vi "SIM Registry Register Node (vector).vi"(0 "Registry In":T1, 5 "Has ZC?":bool, 9 "Output Width":i32=-1, 11 "Input Width":i32=-1, 14 "Tag":string) -> (4 "Registry Out":T1, 6 "Block Idx":i32)   [LabVIEW 2020]
uses:
  <vilib>/Simulation/Implementation/Shared/SIM Registry.llb/SIM Simulation Registry.ctl
  <vilib>/Simulation/Implementation/Shared/SIM Registry.llb/SIM Registry Node Header.ctl
  <vilib>/Simulation/Implementation/Shared/SIM Registry.llb/SIM Registry Node Record.ctl
  <vilib>/Simulation/Implementation/Shared/SIM trigger type.ctl
  <vilib>/Simulation/Implementation/Shared/SIM solver state data.ctl
  <vilib>/Simulation/Implementation/Shared/SIM limit type.ctl
  <vilib>/Simulation/Implementation/Shared/SIM discrete data.ctl
  <vilib>/Simulation/Implementation/Shared/SIM Discrete state data.ctl
  <vilib>/Simulation/Implementation/Shared/SIM Registry.llb/SIM Simulation Registry Error.ctl
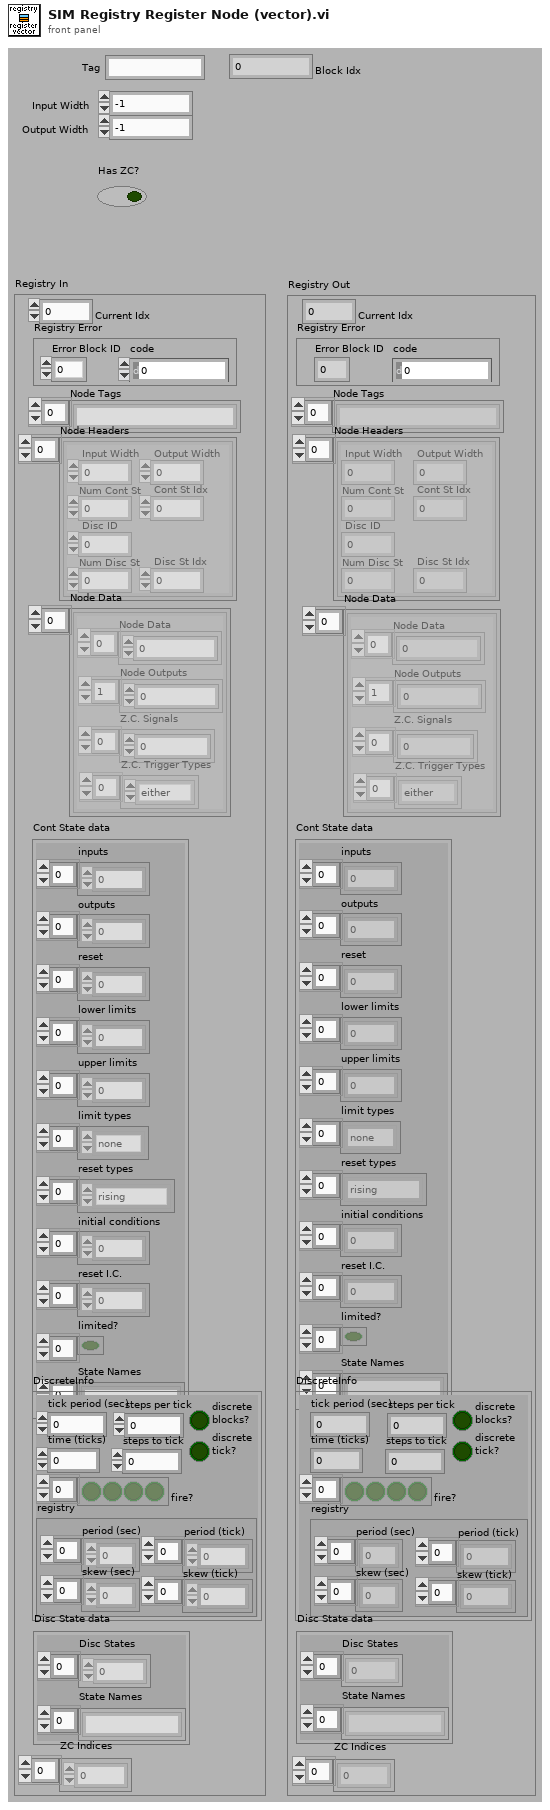
[diagram p1: front panel]
types:
  T1 = typedef "SIM Simulation Registry.ctl" = cluster{"Current Idx":i32, "Node Tags":string[], "Node Headers":T2[], "Node Data":T3[], "Cont State data":T5, "DiscreteInfo":T7, "Disc State data":T8, "Registry Error":T9, "ZC Indices":i32[]}
  T2 = typedef "SIM Registry Node Header.ctl" = cluster{"Input Width":i32, "Disc ID":i32, "Num Cont St":i32, "Cont St Idx":i32, "Num Disc St":i32, "Disc St Idx":i32, "Output Width":i32}
  T3 = typedef "SIM Registry Node Record.ctl" = cluster{"Node Data":dbl[], "Node Outputs":dbl[], "Z.C. Signals":dbl[], "Z.C. Trigger Types":T4[]}
  T4 = typedef "SIM trigger type.ctl" = enum16{"rising", "falling", "either", "none"}
  T5 = typedef "SIM solver state data.ctl" = cluster{"inputs":dbl[], "outputs":dbl[], "reset":dbl[], "lower limits":dbl[], "upper limits":dbl[], "limit types":T6[], "reset types":T4[], "initial conditions":dbl[], "reset I.C.":dbl[], "limited?":bool[], "State Names":string[]}
  T6 = typedef "SIM limit type.ctl" = enum16{"upper", "lower", "both", "none"}
  T7 = typedef "SIM discrete data.ctl" = cluster{"tick period (sec)":dbl, "time (ticks)":i32, "fire?":bool[], "registry":cluster{"period (sec)":dbl[], "skew (sec)":dbl[], "period (tick)":i32[], "skew (tick)":i32[]}, "discrete \nblocks?":bool, "steps per tick":dbl, "steps to tick":dbl, "discrete \ntick?":bool}
  T8 = typedef "SIM Discrete state data.ctl" = cluster{"Disc States":dbl[], "State Names":string[]}
  T9 = typedef "SIM Simulation Registry Error.ctl" = cluster{"Error Block ID":i32, "code":i32}
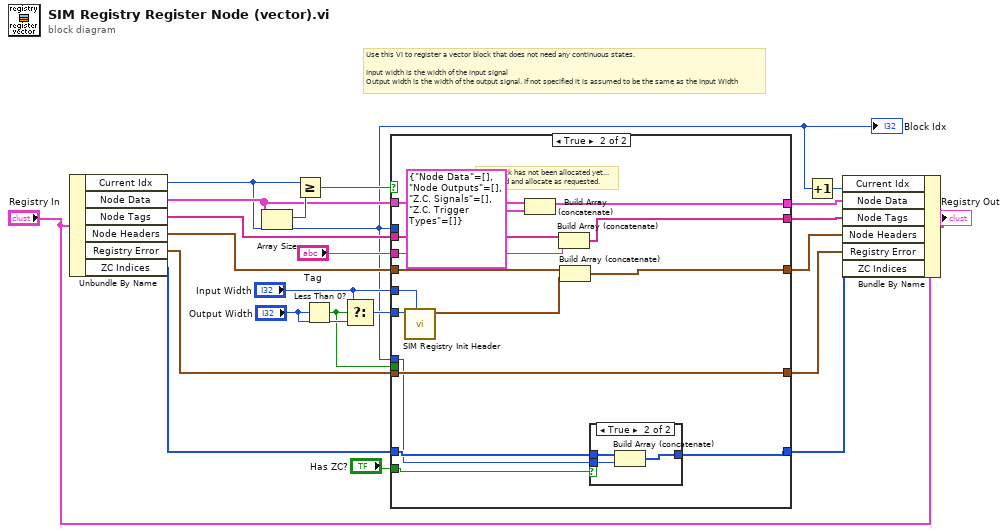
[diagram p0: block diagram]
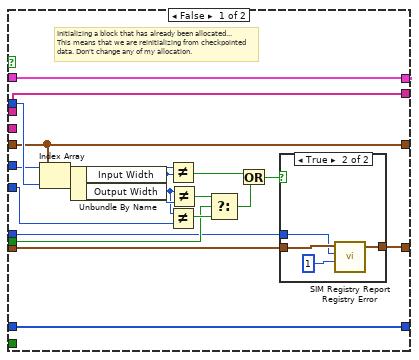
[diagram p2: hidden frame]
diagram:
  # "Use this VI to register a vector block that does not need any continuous states.\n\nInput width is the width of the input signal\nOutput width is the width of the output signal. If not specified it is assumed to be the same as the Input Width"
  n1 = Unbundle By Name("Registry In") -> ("Current Idx"=w5:i32, "Node Data"=w20:T3[], "Node Tags"=w15:string[], "Node Headers"=w13:T2[], "Registry Error"=w8:T9, "ZC Indices"=w2:i32[])
  "Block Idx" <- w5
  n2 = Array Size(array=w20) -> (size(s)=w22:i32)
  n3 = Greater Or Equal?(x=w5, y=w22) -> (x >= y?=w21:bool)
  n4 = Less Than 0?(x="Output Width") -> (x < 0?=w4:bool)
  n5 = Select(t="Input Width", s=w4, f="Output Width") -> (s? t:f=w9:i32)
  n6 = case shown="True" w21 {
    tunnel: w20 -> [w40 w62]
    tunnel: "Tag" -> [_ w59]
    tunnel: [w40 w61] -> w16
    tunnel: w15 -> [w41 w60]
    tunnel: [w41 w57] -> w14
    tunnel: "Input Width" -> [w36 w53]
    tunnel: w5 -> [w39 _]
    tunnel: w13 -> [w37 w56]
    tunnel: [w37 w54] -> w12
    tunnel: w9 -> [w33 w52]
    tunnel: w8 -> [w32 w51]
    tunnel: [w26 w51] -> w7
    tunnel: w5 -> [w24 w49]
    tunnel: w4 -> [w25 _]
    tunnel: [w23 w48] -> w3
    tunnel: w2 -> [w23 w50]
    tunnel: "Has ZC?" -> [_ w47]
    frame False {
      # "Initializing a block that has already been allocated...\nThis means that we are reinitializing from checkpointed\ndata. Don't change any of my allocation."
      n7 = Index Array(array=w37, index=w39) -> (element=w38:T2)
      n8 = Unbundle By Name(w38) -> ("Input Width"=w35:i32, "Output Width"=w34:i32)
      n9 = Not Equal?(x=w36, y=w35) -> (x != y?=w30:bool)
      n10 = Not Equal?(x=w34, y=w33) -> (x != y?=w28:bool)
      n11 = Not Equal?(x=w34, y=w35) -> (x != y?=w29:bool)
      n12 = Select(t=w29, s=w25, f=w28) -> (s? t:f=w27:bool)
      n13 = Or(x=w30, y=w27) -> (x .or. y?=w31:bool)
      n14 = case shown="True" w31 {
        tunnel: w32 -> [w42 w46]
        tunnel: [w42 w45] -> w26
        tunnel: w24 -> [_ w44]
        frame False {
        }
        frame True {
          n15 = call <vilib>:"SIM Registry Report Registry Error.vi"("code"=1, "Block Idx"=w44, "Registry Error"=w46) -> ("Registry Error Out"=w45:T9)  [unwired: 8 out]
        }
      }
    }
    frame True {
      # "This block has not been allocated yet...\nGo ahead and allocate as requested."
      n16 = call <vilib>:"SIM Registry Init Header.vi"("Input Width"=w53, "Output Width"=w52) -> ("Node Header"=w55:T2)  [unwired: 6 in, 3 out]
      n17 = Build Array (concatenate)(w62, T3 {"Node Data"=[], "Node Outputs"=[], "Z.C. Signals"=[], "Z.C. Trigger Types"=[]} ("Node Record")) -> (w61:T3[])
      n18 = Build Array (concatenate)(w60, w59) -> (w57:string[])
      n19 = Build Array (concatenate)(w56, w55) -> (w54:T2[])
      n20 = case shown="True" w47 {
        tunnel: w49 -> [_ w65]
        tunnel: w50 -> [w63 w66]
        tunnel: [w63 w64] -> w48
        frame False {
        }
        frame True {
          n21 = Build Array (concatenate)(w66, w65) -> (w64:i32[])
        }
      }
    }
  }
  n22 = Increment(x=w5) -> (x+1=w11:i32)
  n23 = Bundle By Name(cluster="Registry In", "Current Idx"=w11, "Node Data"=w16, "Node Tags"=w14, "Node Headers"=w12, "Registry Error"=w7, "ZC Indices"=w3) -> (→"Registry Out":T1)
